vi "UT_get section.vi"   [LabVIEW 2020]
uses:
  <vilib>/Utility/Data Type/Get Type Information.vi
  lib/Add clue to error cluster.vi
  lib/TOML to LabVIEW.vi
  <vilib>/addons/_JKI Toolkits/Caraya/classes/Assert/Assert Equal Value and Type_Variant.vi
  <vilib>/addons/_JKI Toolkits/Caraya/classes/Assert/Assert Error.vi
  <vilib>/addons/_JKI Toolkits/Caraya/classes/Assert/Assert Not Error.vi
  lib/TOML.lvlib
  <vilib>/addons/_JKI Toolkits/Caraya/classes/Test/Test.lvclass
  <vilib>/addons/_JKI Toolkits/Caraya/classes/Assert/Assert.lvclass
types:
  T1 = cluster{"string1":string, "string2":string, "string3":string}
  T2 = typedef "TOML.lvlib/TOML Value.ctl" = cluster{"type":enum16{"Table", "Array", "String", "Integer", "Float", "Boolean", "Offset Date-Time", "Local Date-Time", "Local Date", "Local Time", "Path"}, "value":variant}
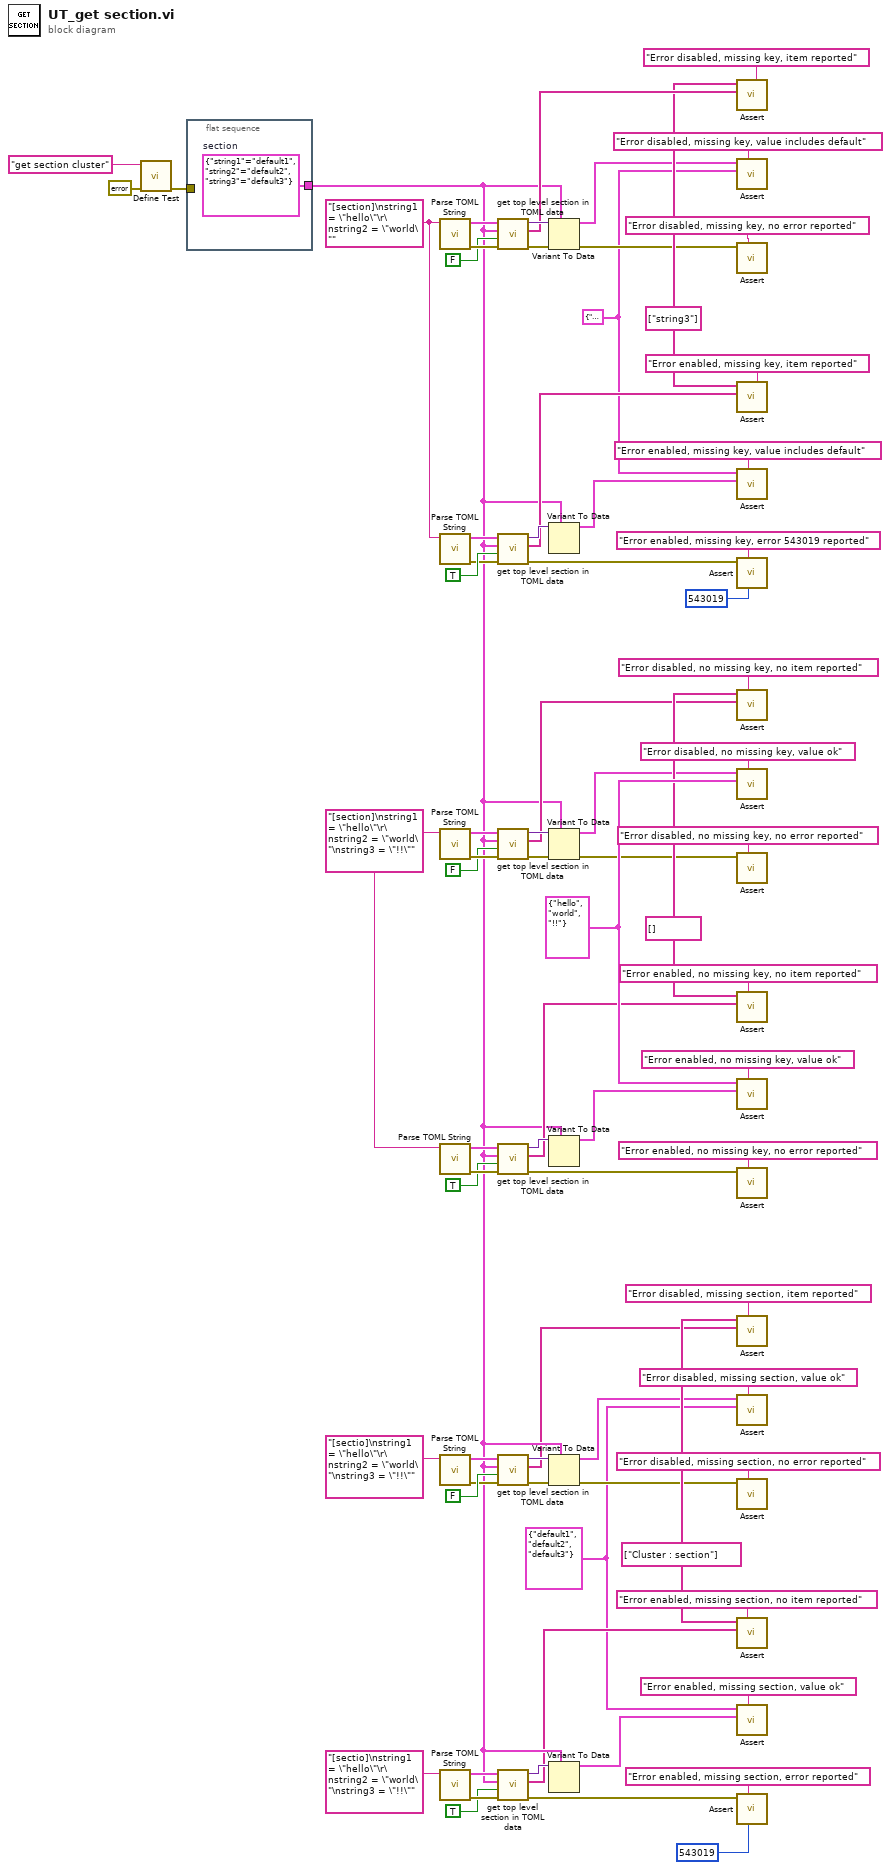
[diagram p0: block diagram]
diagram:
  w2 = T1 {"string1"="default1", "string2"="default2", "string3"="default3"} ("data")
  w12 = string[] ["Cluster : section"] ("Missing elements")
  w41 = T1 {"string1"="hello", "string2"="world", "string3"="!!"} ("data")
  w37 = string[] [] ("Missing elements")
  w42 = T1 {"string1"="hello", "string2"="world", "string3"="default3"} ("data")
  w50 = string[] ["string3"] ("Missing elements")
  w61 = "[section]\nstring1 = \"hello\"\r\nstring2 = \"world\"\nstring3 = \"!!\"" ("x")
  w66 = "[section]\nstring1 = \"hello\"\r\nstring2 = \"world\"" ("x")
  n1 = call <vilib>:"Define Test.vi"("error in (no error)"=errorcluster {"status"=FALSE, "code"=0, "source"=""}, "Label (VI Title)"="get section cluster") -> ("error out"=w58:errorcluster)  [unwired: 8 in, 1 out]
  n2 = flat-sequence {
    tunnel: [w80] -> w16
    tunnel: w58 -> [_]
    frame #0 {
      w80 = T1 {"string1"="default1", "string2"="default2", "string3"="default3"}  # section
    }
  }
  n3 = call "Parse TOML String.vi"("String"=w66) -> ("error out"=w77:errorcluster, "Value"=w78:T2)  [unwired: 9 in]
  n4 = call "Parse TOML String.vi"("String"=w66) -> ("error out"=w69:errorcluster, "Value"=w68:T2)  [unwired: 9 in]
  n5 = call "Parse TOML String.vi"("String"=w61) -> ("error out"=w76:errorcluster, "Value"=w75:T2)  [unwired: 9 in]
  n6 = call "Parse TOML String.vi"("String"=w61) -> ("error out"=w63:errorcluster, "Value"=w64:T2)  [unwired: 9 in]
  n7 = call "Parse TOML String.vi"("String"="[sectio]\nstring1 = \"hello\"\r\nstring2 = \"world\"\nstring3 = \"!!\"" ("x")) -> ("error out"=w22:errorcluster, "Value"=w23:T2)  [unwired: 9 in]
  n8 = call "Parse TOML String.vi"("String"="[sectio]\nstring1 = \"hello\"\r\nstring2 = \"world\"\nstring3 = \"!!\"" ("x")) -> ("error out"=w21:errorcluster, "Value"=w20:T2)  [unwired: 9 in]
  n9 = call "get top level section in TOML data.vi"("error in (no error)"=w77, "Error if missing element"=FALSE, "Section datatype"=w16, "Value in"=w78) -> ("error out"=w46:errorcluster, "Missing elements"=w51:string[], "LV Value"=w79:variant)  [unwired: 5 in]
  n10 = call "get top level section in TOML data.vi"("error in (no error)"=w69, "Error if missing element"=TRUE, "Section datatype"=w16, "Value in"=w68) -> ("error out"=w53:errorcluster, "Missing elements"=w55:string[], "LV Value"=w67:variant)  [unwired: 5 in]
  n11 = call "get top level section in TOML data.vi"("error in (no error)"=w76, "Error if missing element"=FALSE, "Section datatype"=w16, "Value in"=w75) -> ("error out"=w73:errorcluster, "Missing elements"=w28:string[], "LV Value"=w74:variant)  [unwired: 5 in]
  n12 = call "get top level section in TOML data.vi"("error in (no error)"=w63, "Error if missing element"=TRUE, "Section datatype"=w16, "Value in"=w64) -> ("error out"=w32:errorcluster, "Missing elements"=w30:string[], "LV Value"=w65:variant)  [unwired: 5 in]
  n13 = call "get top level section in TOML data.vi"("error in (no error)"=w22, "Error if missing element"=FALSE, "Section datatype"=w16, "Value in"=w23) -> ("error out"=w25:errorcluster, "Missing elements"=w3:string[], "LV Value"=w24:variant)  [unwired: 5 in]
  n14 = call "get top level section in TOML data.vi"("error in (no error)"=w21, "Error if missing element"=TRUE, "Section datatype"=w16, "Value in"=w20) -> ("error out"=w8:errorcluster, "Missing elements"=w5:string[], "LV Value"=w19:variant)  [unwired: 5 in]
  n15 = Variant To Data(error in=w46, type=w16, Variant=w79) -> (data=w43:T1, error out=w44:errorcluster)
  n16 = Variant To Data(type=w16, Variant=w67) -> (data=w47:T1)  [unwired: 1 in, 1 out]
  n17 = Variant To Data(error in=w73, type=w16, Variant=w74) -> (data=w29:T1, error out=w33:errorcluster)
  n18 = Variant To Data(type=w16, Variant=w65) -> (data=w31:T1)  [unwired: 1 in, 1 out]
  n19 = Variant To Data(error in=w25, type=w16, Variant=w24) -> (data=w4:T1, error out=w7:errorcluster)
  n20 = Variant To Data(type=w16, Variant=w19) -> (data=w6:T1)  [unwired: 1 in, 1 out]
  n21 = call-poly <vilib>:"Assert.vi"("Label"="Error disabled, missing key, item reported" ("Label (VI Title)"), "Y"=w51, "X"=w50) -> ()  [unwired: 7 in, 2 out]
  n22 = call-poly <vilib>:"Assert.vi"("Label"="Error disabled, missing key, value includes default" ("Label (VI Title)"), "Y"=w42, "X"=w43) -> ()  [unwired: 7 in, 2 out]
  n23 = call-poly <vilib>:"Assert.vi"("Label"="Error disabled, missing key, no error reported" ("Label (VI Title)"), "Not Error?"=w44) -> ()  [unwired: 8 in, 2 out]
  n24 = call-poly <vilib>:"Assert.vi"("Label"="Error enabled, missing key, item reported" ("Label (VI Title)"), "Y"=w55, "X"=w50) -> ()  [unwired: 7 in, 2 out]
  n25 = call-poly <vilib>:"Assert.vi"("Label"="Error enabled, missing key, value includes default" ("Label (VI Title)"), "Y"=w47, "X"=w42) -> ()  [unwired: 7 in, 2 out]
  n26 = call-poly <vilib>:"Assert.vi"("error code (1)"=543019, "Label"="Error enabled, missing key, error 543019 reported" ("Label (VI Title)"), "Error?"=w53) -> ()  [unwired: 7 in, 2 out]
  n27 = call-poly <vilib>:"Assert.vi"("Label"="Error disabled, no missing key, no item reported" ("Label (VI Title)"), "Y"=w28, "X"=w37) -> ()  [unwired: 7 in, 2 out]
  n28 = call-poly <vilib>:"Assert.vi"("Label"="Error disabled, no missing key, value ok" ("Label (VI Title)"), "Y"=w41, "X"=w29) -> ()  [unwired: 7 in, 2 out]
  n29 = call-poly <vilib>:"Assert.vi"("Label"="Error disabled, no missing key, no error reported" ("Label (VI Title)"), "Not Error?"=w33) -> ()  [unwired: 8 in, 2 out]
  n30 = call-poly <vilib>:"Assert.vi"("Label"="Error enabled, no missing key, no item reported" ("Label (VI Title)"), "Y"=w30, "X"=w37) -> ()  [unwired: 7 in, 2 out]
  n31 = call-poly <vilib>:"Assert.vi"("Label"="Error enabled, no missing key, value ok" ("Label (VI Title)"), "Y"=w31, "X"=w41) -> ()  [unwired: 7 in, 2 out]
  n32 = call-poly <vilib>:"Assert.vi"("Label"="Error enabled, no missing key, no error reported" ("Label (VI Title)"), "Not Error?"=w32) -> ()  [unwired: 8 in, 2 out]
  n33 = call-poly <vilib>:"Assert.vi"("Label"="Error disabled, missing section, item reported" ("Label (VI Title)"), "Y"=w3, "X"=w12) -> ()  [unwired: 7 in, 2 out]
  n34 = call-poly <vilib>:"Assert.vi"("Label"="Error disabled, missing section, value ok" ("Label (VI Title)"), "Y"=w2, "X"=w4) -> ()  [unwired: 7 in, 2 out]
  n35 = call-poly <vilib>:"Assert.vi"("Label"="Error disabled, missing section, no error reported" ("Label (VI Title)"), "Not Error?"=w7) -> ()  [unwired: 8 in, 2 out]
  n36 = call-poly <vilib>:"Assert.vi"("Label"="Error enabled, missing section, no item reported" ("Label (VI Title)"), "Y"=w5, "X"=w12) -> ()  [unwired: 7 in, 2 out]
  n37 = call-poly <vilib>:"Assert.vi"("Label"="Error enabled, missing section, value ok" ("Label (VI Title)"), "Y"=w6, "X"=w2) -> ()  [unwired: 7 in, 2 out]
  n38 = call-poly <vilib>:"Assert.vi"("error code (1)"=543019, "Label"="Error enabled, missing section, error reported" ("Label (VI Title)"), "Error?"=w8) -> ()  [unwired: 7 in, 2 out]
